vi "fg-Overlay images interface.vi"(6 "Function":T1, 8 "error in (no error)":errorcluster) -> (0 "error out":errorcluster, 1 "GreenPOIMax":T2, 2 "RedPOIMax":T2)   [LabVIEW 2017]
uses:
  <vilib>/vision/Image Controls.llb/IMAQ Image.ctl
  Typedefs/Overlay FG functions.ctl
  Global variables/gl_Functional Imaging-Global variables.vi
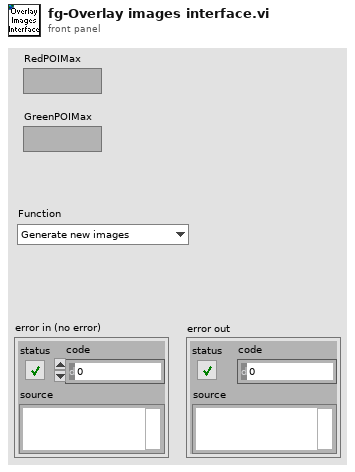
[diagram p1: front panel]
types:
  T1 = typedef "Overlay FG functions.ctl" = enum16{"Generate new images", "Get stored images", "Clear"}
  T2 = typedef "IMAQ Image.ctl" = refnum<image>
  T3 = typedef "Functional Imging UI Refs.ctl" = cluster{"Menu ref":refnum<k9>, "Image control":refnum<vi>, "VI ref":refnum<vi>, "XGrapher":refnum<vi>, "Smoothing":refnum<vi>, "POI Averaging":refnum<vi>, "Normalize":refnum<vi>, "POI data points in each trial":refnum<vi>, "Channel":refnum<vi>, "Experiment data folder path":refnum<vi>, "[ROI vis]":refnum<vi>, "[Groups] visbl":T4, "Group Name":refnum<vi>, "POI index":refnum<vi>, "Trial No.":refnum<vi>, "Intensity Zoom":refnum<vi>, "Trial Cursor Enabled":refnum<vi>, "Number of Trials (ind 1)":refnum<vi>, "Number of Trials (ind 2)":refnum<vi>, "MiniScans Available":refnum<vi>, "POI Available":refnum<vi>, "Defer graph updates":refnum<vi>, "Waveform selector":refnum<vi>, "#of selected POI":refnum<vi>, "#of selected MiniScans":refnum<vi>, "#of selected groups":refnum<vi>, "Max Z-Projection":refnum<vi>, "Z-Plane Selector":refnum<vi>, "Index of miniscan point to visualise":refnum<vi>, "ROI vis. mode":refnum<vi>, "Total # of points":refnum<vi>, "Index of group clicked on":refnum<vi>, "Pane 1":refnum<vi>, "Pane 2":refnum<vi>, "Pane 3":refnum<vi>, "Pane 4":refnum<vi>, "Pane 5":refnum<vi>, "Pane 6":refnum<vi>, "Deselect all ROI":refnum<vi>, "Deselect all groups":refnum<vi>}
  T4 = typedef "Groups array referecne.ctl" = refnum<vi>
  T5 = typedef "ROI selector array.ctl" = T6[]
  T6 = typedef "Interface-ROI selection cluster.ctl" = cluster{"ROI number":i32, "ROI ID":T7, "Visibility":bool}
  T7 = typedef "ROI ID Enum.ctl" = enum16{"Point", "MiniScan", "Comp. MiniScan", "Rectangle", "Comp. volume", "Arb. plane point"}
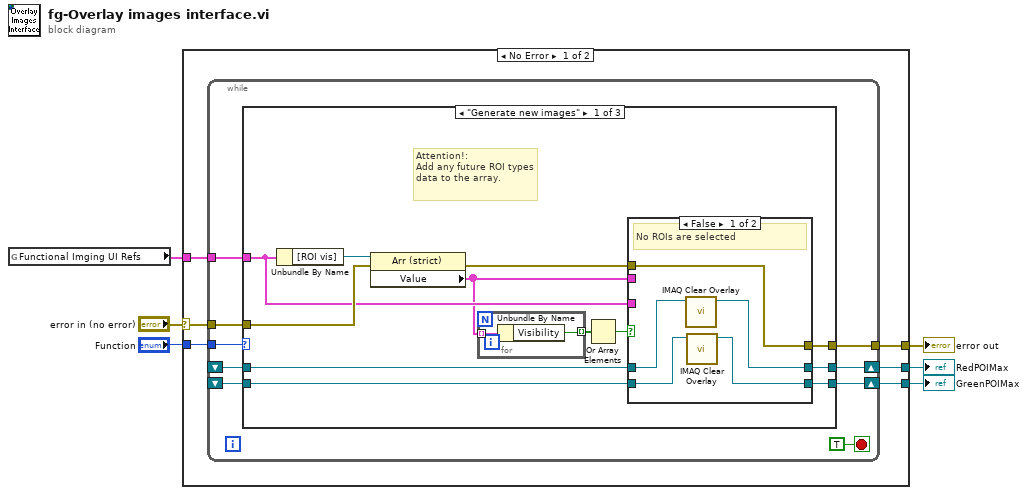
[diagram p0: block diagram]
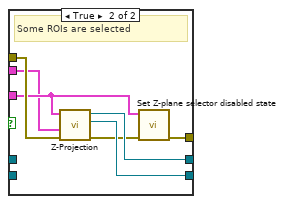
[diagram p2: hidden frame]
diagram:
  n1 = global read "gl_Functional Imaging-Global variables.vi" "Functional Imging UI Refs"() -> (w1:T3)
  n2 = case shown="No Error" "error in (no error)" {
    selector: "error in (no error)" -> [w7 w52]
    tunnel: [w12 w52] -> w6
    tunnel: [w11 _] -> w5
    tunnel: [w10 _] -> w4
    tunnel: w1 -> [w9 _]
    tunnel: "Function" -> [w8 _]
    frame No Error {
      n3 = while {
        tunnel: [w21] -> w12
        tunnel: w9 -> [w18]
        shift-right: [w19] -> w10
        shift-left: _ -> [w16]
        shift-right: [w20] -> w11
        shift-left: _ -> [w15]
        tunnel: w8 -> [w14]
        tunnel: w7 -> [w13]
        stop <- TRUE stop-if-true
        n4 = case shown="\"Generate new images\"" w14 {
          tunnel: [w28 w48 w51] -> w21
          tunnel: [w32 w49 _] -> w20
          tunnel: [w31 w50 _] -> w19
          tunnel: w18 -> [w27 _ _]
          tunnel: w16 -> [w26 w50 _]
          tunnel: w15 -> [w25 w49 _]
          tunnel: w13 -> [w29 w48 w51]
          frame "Generate new images" {
            # "Attention!:\nAdd any future ROI types data to the array."
            n5 = Unbundle By Name(w27) -> ("[ROI vis]"=w33:refnum<vi>)
            n6 = property on="Property Node" class="Arr (strict)"(reference=w33, error in=w29) -> (error out=w30:errorcluster, "Value"=w24:T5)  [unwired: 1 out]
            n7 = for {
              tunnel: w24 -> [w35] mode=indexing
              tunnel: [w34] -> w23 mode=indexing
              n8 = Unbundle By Name(w35) -> ("Visibility"=w34:bool)
            }
            n9 = Or Array Elements(Boolean array=w23) -> (logical OR=w22:bool)
            n10 = case shown="False" w22 {
              tunnel: [w36 w47] -> w32
              tunnel: [w38 w46] -> w31
              tunnel: w30 -> [w40 w45]
              tunnel: [w40 w43] -> w28
              tunnel: w27 -> [_ w42]
              tunnel: w24 -> [_ w41]
              tunnel: w26 -> [w39 _]
              tunnel: w25 -> [w37 _]
              frame False {
                # "No ROIs are selected"
                n11 = call "IMAQ Clear Overlay"("Image"=w39) -> ("Image Out"=w38:T2)  [unwired: 9 in, 1 out]
                n12 = call "IMAQ Clear Overlay"("Image"=w37) -> ("Image Out"=w36:T2)  [unwired: 9 in, 1 out]
              }
              frame True {
                # "Some ROIs are selected"
                n13 = call "Z-Projection.vi"("error in"=w45, "[ROI vis]"=w41, "Functional Imging UI Refs"=w42) -> ("error out"=w44:errorcluster, "GreenPOIMax"=w47:T2, "RedPOIMax"=w46:T2)  [unwired: 6 in]
                n14 = call "Set Z-plane selector disabled state.vi"("error in (no error)"=w44, "Functional Imging UI Refs"=w42) -> ("error out"=w43:errorcluster)  [unwired: 9 in]
              }
            }
          }
          frame "Get stored images", Default {
          }
          frame "Clear" {
          }
        }
      }
    }
    frame Error {
    }
  }
  "error out" <- w6
  "GreenPOIMax" <- w5
  "RedPOIMax" <- w4
